vi "Ch_data_title_pattern (SubVI).vi"(9 "Единица измерений":string) -> (0 "error out":errorcluster, 2 "Path":path, 3 "Byte Stream File out":refnum<file>, 6 "cancelled":bool)   [LabVIEW 2015]
panel:
  in  "error in":errorcluster
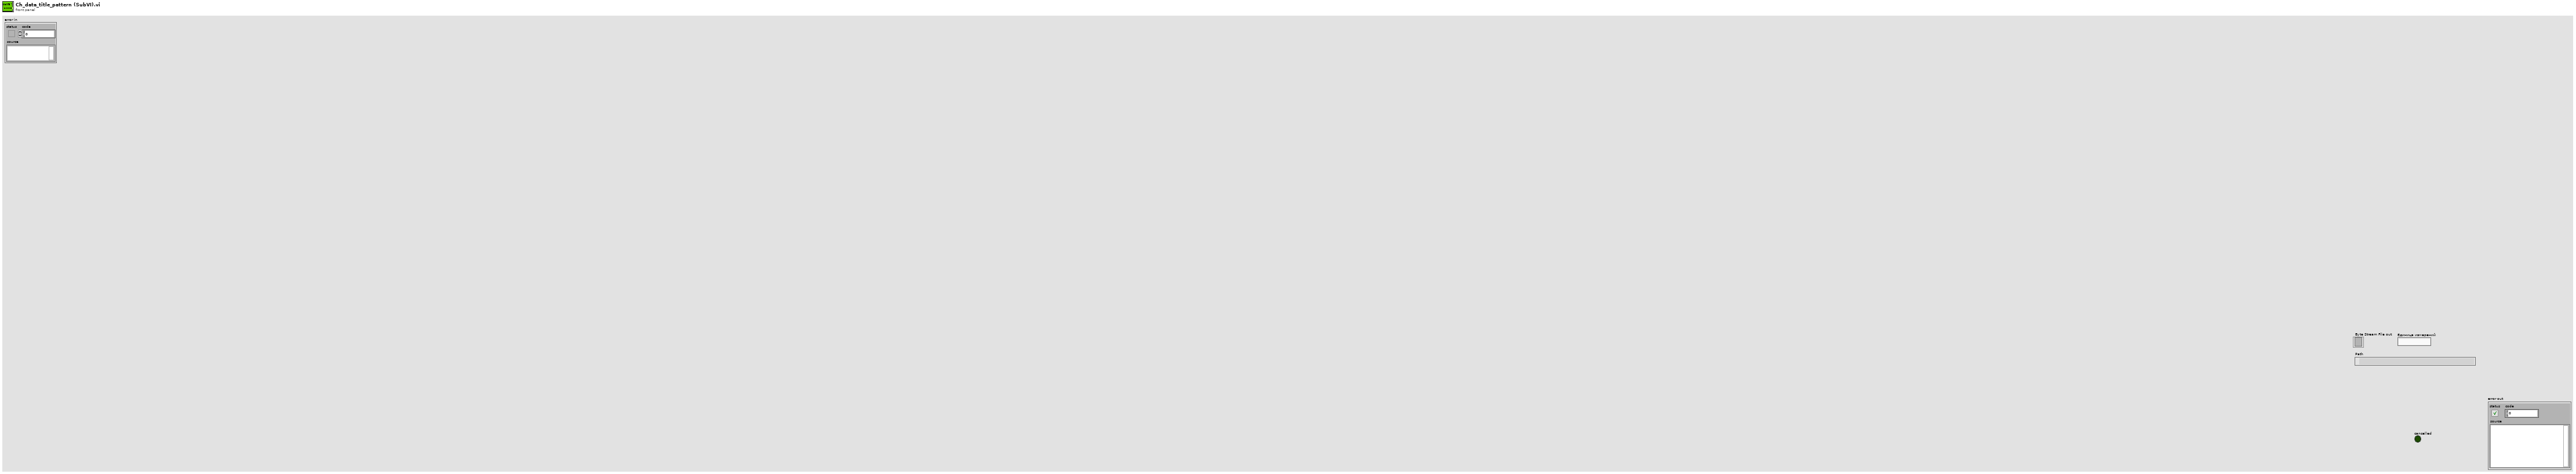
[diagram p1: front panel]
types:
  T1 = enum16{"open", "replace", "create", "open or create", "replace or create", "replace or create with confirmation"}
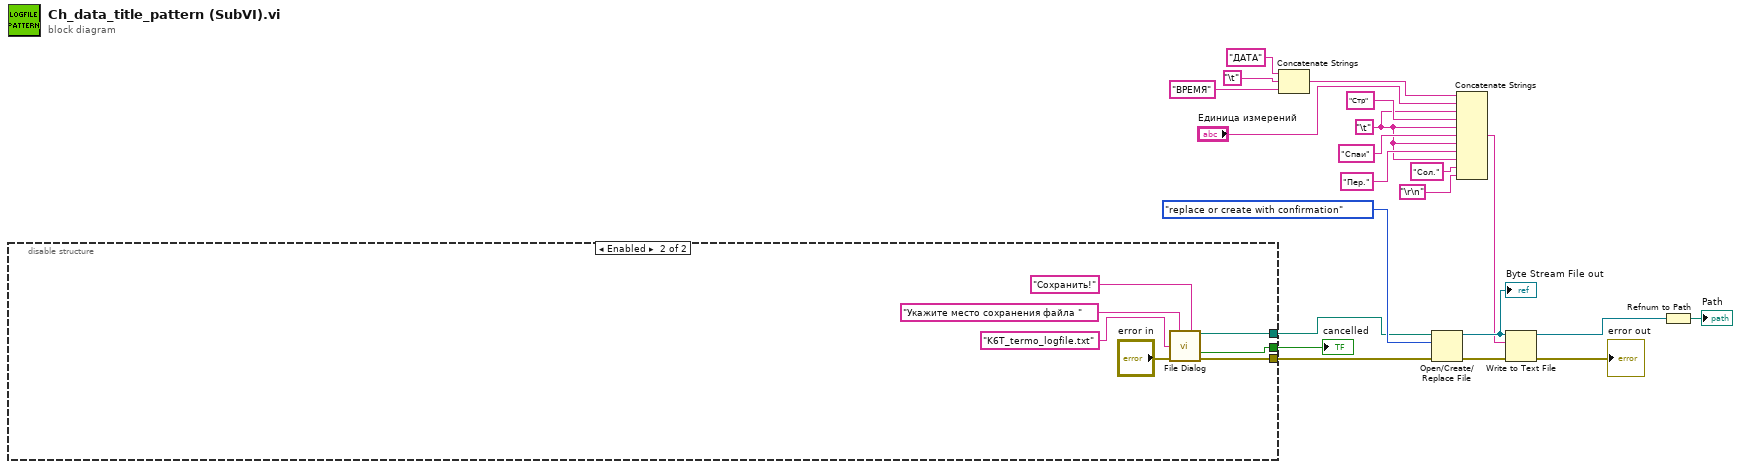
[diagram p0: block diagram]
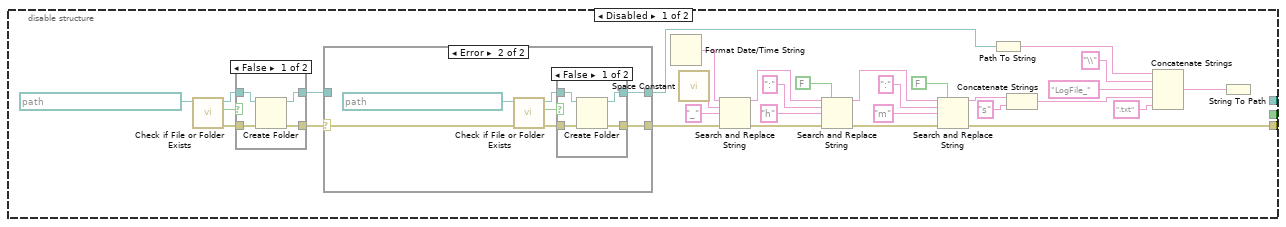
[diagram p2: hidden frame]
diagram:
  w11 = "\t"
  n1 = disable-structure shown="Enabled" {
    disable-tunnel: [w29 w76] -> w15
    disable-tunnel: [_ w75] -> w2
    disable-tunnel: [_ w74] -> w1
    frame Disabled {
      n2 = call <vilib>:"Check if File or Folder Exists.vi"("path"=path "D:/Лог-файл термометрии" ("path (use dialog)")) -> ("error out"=w27:errorcluster, "file or folder exists?"=w25:bool, "dup path"=w28:path, "error in (no error)"=w26:errorcluster)  [unwired: 7 out]
      n3 = case shown="False" w25 {
        tunnel: [w71 w73] -> w23
        tunnel: w28 -> [w70 w73]
        tunnel: w27 -> [w69 w72]
        tunnel: [w68 w72] -> w24
        frame False {
          n4 = Create Folder(path (use dialog)=w70, error in=w69) -> (created path=w71:path, error out=w68:errorcluster)  [unwired: 2 out]
        }
        frame True {
        }
      }
      n5 = case shown="Error" w24 {
        selector: w24 -> [w53 w55]
        tunnel: w23 -> [w54 _]
        tunnel: [w54 w58] -> w30
        tunnel: [w53 w57] -> w31
        frame No Error {
        }
        frame Error {
          n6 = call <vilib>:"Check if File or Folder Exists.vi"("error in (no error)"=w55, "path"=path "E:/Лог-файл термометрии" ("path (use dialog)")) -> ("error out"=w60:errorcluster, "file or folder exists?"=w59:bool, "dup path"=w61:path)  [unwired: 7 out]
          n7 = case shown="False" w59 {
            tunnel: [w65 w67] -> w58
            tunnel: w61 -> [w64 w67]
            tunnel: w60 -> [w63 w66]
            tunnel: [w62 w66] -> w57
            frame False {
              n8 = Create Folder(path (use dialog)=w64, error in=w63) -> (created path=w65:path, error out=w62:errorcluster)  [unwired: 2 out]
            }
            frame True {
            }
          }
        }
      }
      n9 = Format Date/Time String() -> (date/time string=w52:string)  [unwired: 3 out]
      n10 = call <vilib>:"Space Constant.vi"() -> ("String"=w33:string)
      n11 = Search and Replace String(input string=w52, search string=w33, replace string="_" ("replace string (\"\")"), error in=w31) -> (result string=w35:string, error out=w45:errorcluster)  [unwired: 6 out]
      n12 = Search and Replace String(replace all?=FALSE ("replace all? (F)"), input string=w35, search string=":", replace string="h" ("replace string (\"\")"), error in=w45) -> (result string=w42:string, error out=w46:errorcluster)  [unwired: 5 out]
      n13 = Search and Replace String(replace all?=FALSE ("replace all? (F)"), input string=w42, search string=":", replace string="m" ("replace string (\"\")"), error in=w46) -> (result string=w47:string, error out=w29:errorcluster)  [unwired: 5 out]
      n14 = Path To String(path=w30) -> (string=w43:string)
      n15 = Concatenate Strings(w47, "s" ("string")) -> (w50:string)
      n16 = Concatenate Strings(w43, "\\" ("string"), "LogFile_" ("string"), w50, ".txt" ("default name")) -> (w32:string)
      n17 = String To Path(string=w32) -> ()  [unwired: 1 out]
    }
    frame Enabled {
      n18 = call "File Dialog"("prompt"="Укажите место сохранения файла " ("string"), "button label"="Сохранить!" ("string"), "default name"="K6T_termo_logfile.txt" ("string"), "error in"="error in") -> ("selected path"=w75:path, "cancelled"=w74:bool, "error out"=w76:errorcluster)  [unwired: 8 in, 1 out]
    }
  }
  "cancelled" <- w1
  n19 = Concatenate Strings("ДАТА" ("string"), "\t", "ВРЕМЯ" ("string")) -> (w5:string)
  n20 = Open/Create/Replace File(file path (use dialog)=w2, error in=w15, operation (0:open)=T1."replace or create with confirmation") -> (refnum out=w20:refnum<file>, error out=w18:errorcluster)  [unwired: 4 out]
  "Byte Stream File out" <- w20
  n21 = Concatenate Strings(w5, "Единица измерений", w11, "Стр" ("string"), w11, "Спаи" ("string"), w11, "Пер." ("string"), w11, "Сол." ("string"), "\r\n") -> (w17:string)
  n22 = Write to Text File(file (use dialog)=w20, text=w17, error in=w18) -> (refnum out=w4:refnum<file>, error out=→"error out":errorcluster)  [unwired: 2 out]
  n23 = Refnum to Path(1:w4) -> (0:→"Path":path)
